vi "Read UI references.vi"(8 "error in (no error)":errorcluster, 11 "Data in":refnum<class "Data.lvclass">) -> (0 "error out":errorcluster, 2 "UI references":T1, 3 "Data out":refnum<class "Data.lvclass">)   [LabVIEW 2018, in "Tracker Main.lvlib" / "Data.lvclass"]
uses:
  Data.lvclass
  SubVi's/Controls/CTL_All_References_2.ctl
  Common/Typedefs/CTL_Panes_and_VIs_References.ctl
  Common/Typedefs/CTL_Indicators_References_2.ctl
  Common/Typedefs/CTL_Controls_References_2.ctl
  Data.lvclass/Data.ctl
  Common_Resources.lvlib
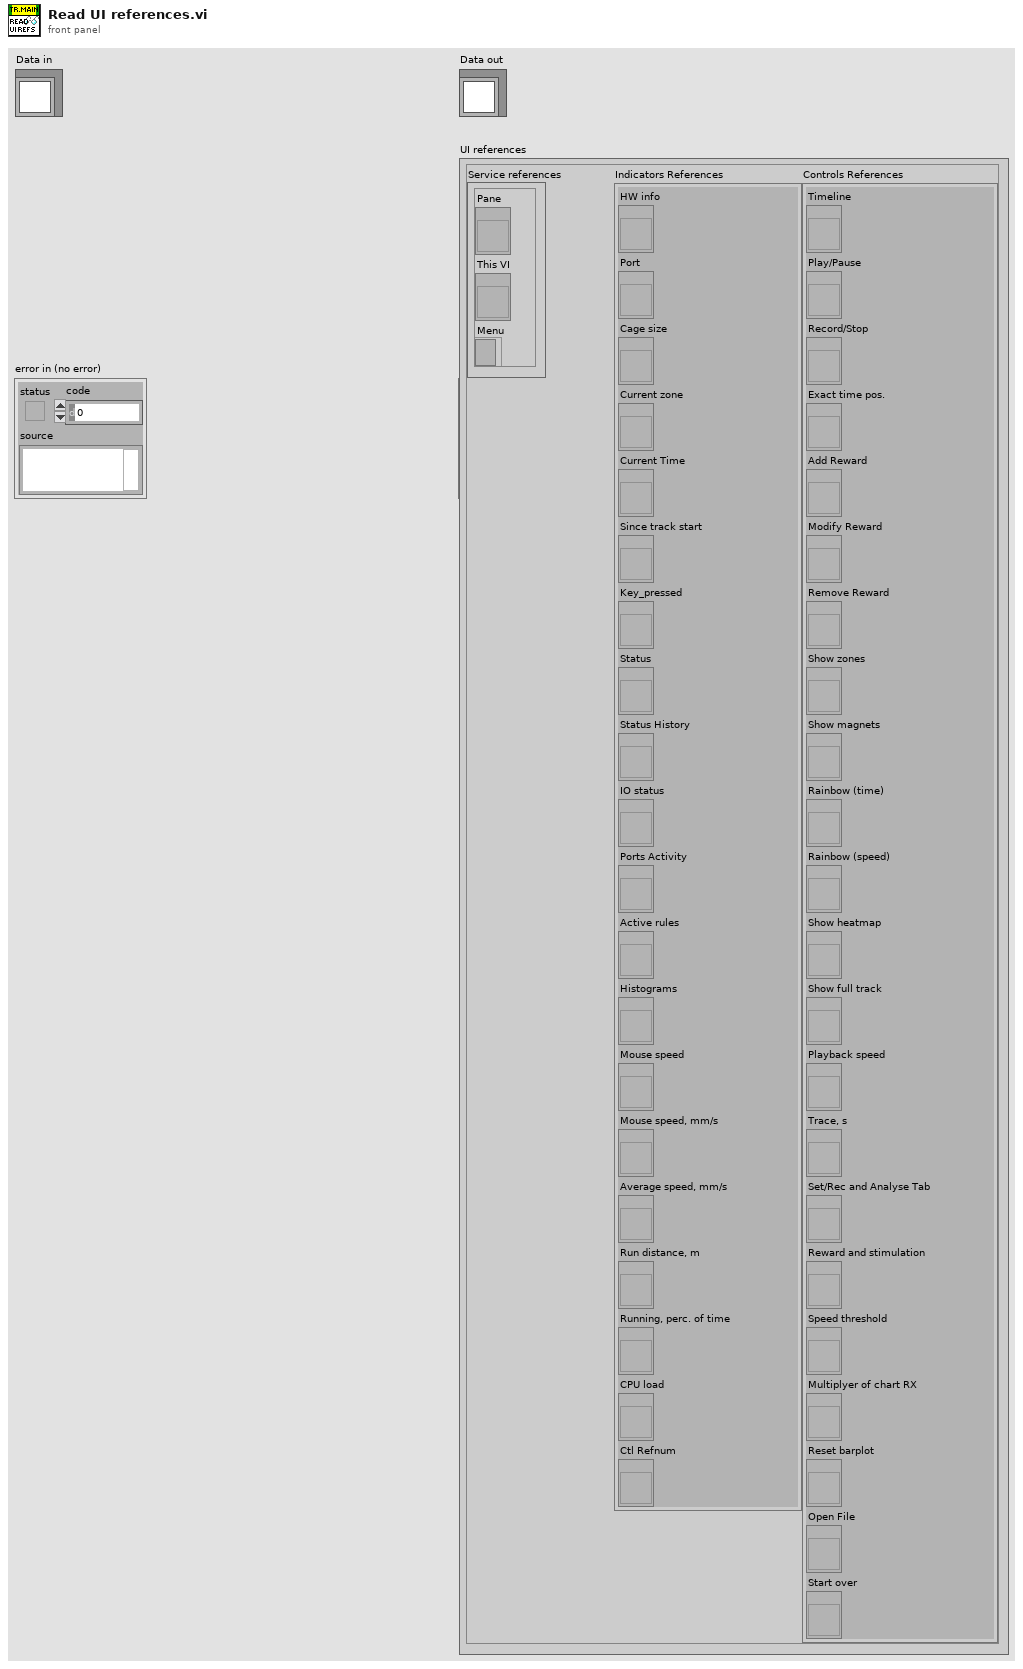
[diagram p1: front panel]
types:
  T1 = typedef "Common_Resources.lvlib/CTL_All_References_2.ctl" = cluster{"Service references":T2, "Indicators References":T3, "Controls References":T4}
  T2 = typedef "Common_Resources.lvlib/CTL_Panes_and_VIs_References.ctl" = cluster{"Pane":refnum<vi>, "This VI":refnum<vi>, "Menu":refnum<k9>}
  T3 = typedef "Common_Resources.lvlib/CTL_Indicators_References_2.ctl" = cluster{"HW info":refnum<vi>, "Port":refnum<vi>, "Cage size":refnum<vi>, "Current zone":refnum<vi>, "Current Time":refnum<vi>, "Since track start":refnum<vi>, "Key_pressed":refnum<vi>, "Status":refnum<vi>, "Status History":refnum<vi>, "IO status":refnum<vi>, "Ports Activity":refnum<vi>, "Active rules":refnum<vi>, "Histograms":refnum<vi>, "Mouse speed":refnum<vi>, "Mouse speed, mm/s":refnum<vi>, "Average speed, mm/s":refnum<vi>, "Run distance, m":refnum<vi>, "Running, perc. of time":refnum<vi>, "CPU load":refnum<vi>, "Ctl Refnum":refnum<vi>}
  T4 = typedef "Common_Resources.lvlib/CTL_Controls_References_2.ctl" = cluster{"Timeline":refnum<vi>, "Play/Pause":refnum<vi>, "Record/Stop":refnum<vi>, "Exact time pos.":refnum<vi>, "Add Reward":refnum<vi>, "Modify Reward":refnum<vi>, "Remove Reward":refnum<vi>, "Show zones":refnum<vi>, "Show magnets":refnum<vi>, "Rainbow (time)":refnum<vi>, "Rainbow (speed)":refnum<vi>, "Show heatmap":refnum<vi>, "Show full track":refnum<vi>, "Playback speed":refnum<vi>, "Trace, s":refnum<vi>, "Set/Rec and Analyse Tab":refnum<vi>, "Reward and stimulation":refnum<vi>, "Speed threshold":refnum<vi>, "Multiplyer of chart RX":refnum<vi>, "Reset barplot":refnum<vi>, "Open File":refnum<vi>, "Start over":refnum<vi>}
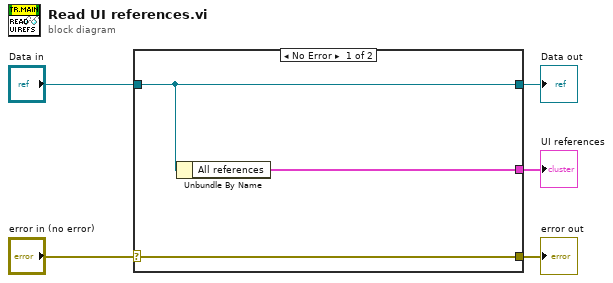
[diagram p0: block diagram]
diagram:
  n1 = case shown="No Error" "error in (no error)" {
    selector: "error in (no error)" -> [w8 w9]
    tunnel: [w8 w9] -> w4
    tunnel: [w7 w10] -> w2
    tunnel: "Data in" -> [w7 w10]
    tunnel: [w6 _] -> w1
    frame No Error {
      n2 = Unbundle By Name(w7) -> ("All references"=w6:T1)
    }
    frame Error {
    }
  }
  "error out" <- w4
  "Data out" <- w2
  "UI references" <- w1
